vi "WL_XNET_GetDBCInfo.vi"(8 "err in":errorcluster caption="error") -> (0 "err out":errorcluster caption="error", 3 "DBC Settings":T1={"ByteOrder"=[enum."Motorola", enum."Motorola"], "Type"=[], "Factor"=[1.0, 1.0], "Offset"=[0.0, 0.0], "Startbit"=[27, 43], "Length"=[16, 16], "Mux"=[FALSE, FALSE], "Name"=["", ""]} {"Offset" format="%.3f"; "Factor" format="%.3f"})   [LabVIEW 2021]
uses:
  <vilib>/xnet/xnet.llb/XNET Database Close (Signal).vi
  <vilib>/xnet/xnet.llb/XNET Database Close (Cluster).vi
  <vilib>/xnet/xnet.llb/XNET Database Close (Database).vi
  WL_XNET_Globals.vi
  <resource>/objmgr/xnet.rc
panel:
  out "MuxDynamic":bool[](array[boolean])
  out "Mux":bool[](array[boolean])
  in  "default baud rate (0)":u64=500000
  in  "CAN DBC":path=path "G:/07_GLOBE/00_git/XLP80/02_Documentation/Daten Albert_10-08-2022/Globe_CAN_500_2022-08-08_v26.dbc"
  out "Frame":string[](array[string])
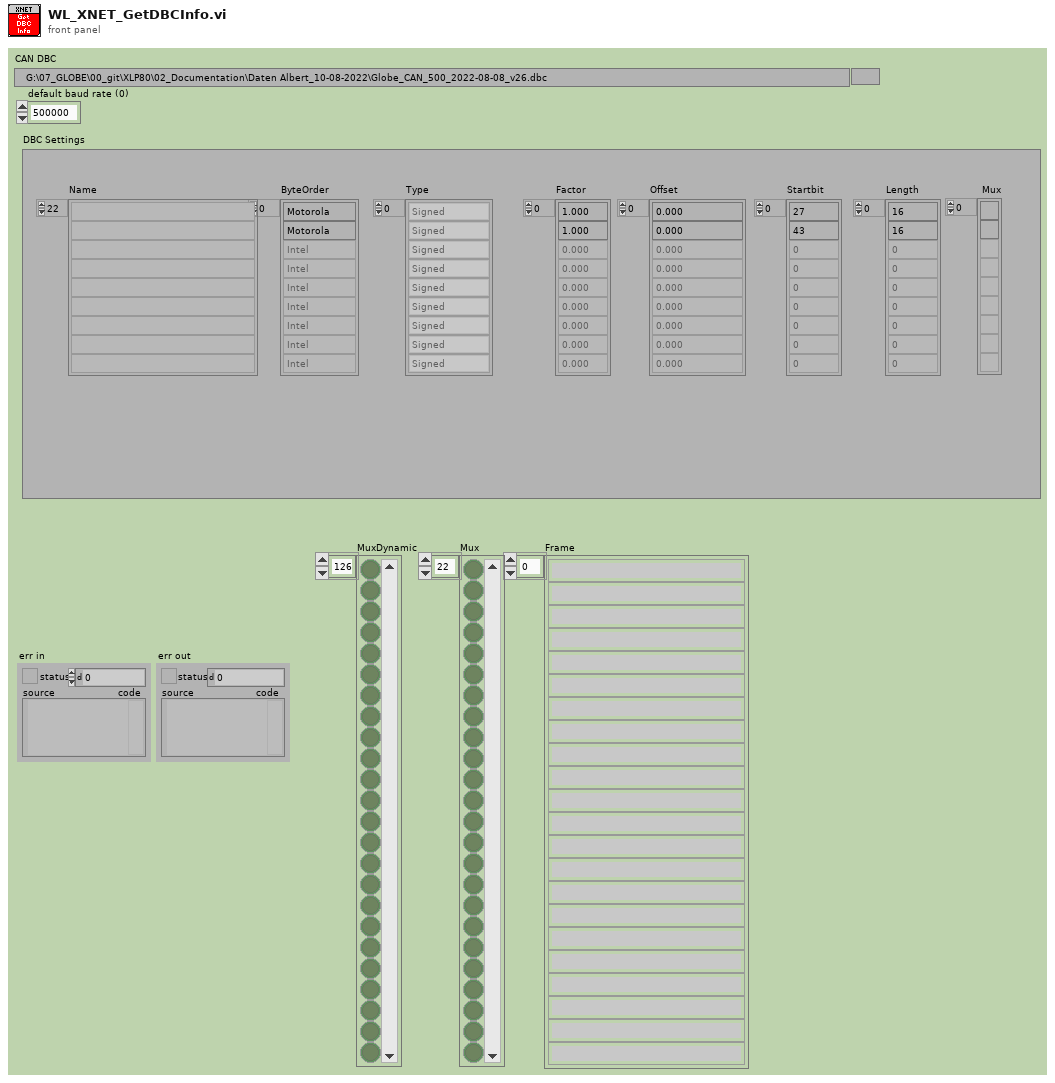
[diagram p1: front panel]
types:
  T1 = cluster{"ByteOrder":enum16{"Intel", "Motorola"}[], "Type":enum16{"Signed", "Unsigned", "IEEE Float", "Byte Array"}[], "Factor":dbl[], "Offset":dbl[], "Startbit":u32[], "Length":u32[], "Mux":bool[], "Name":string[]}
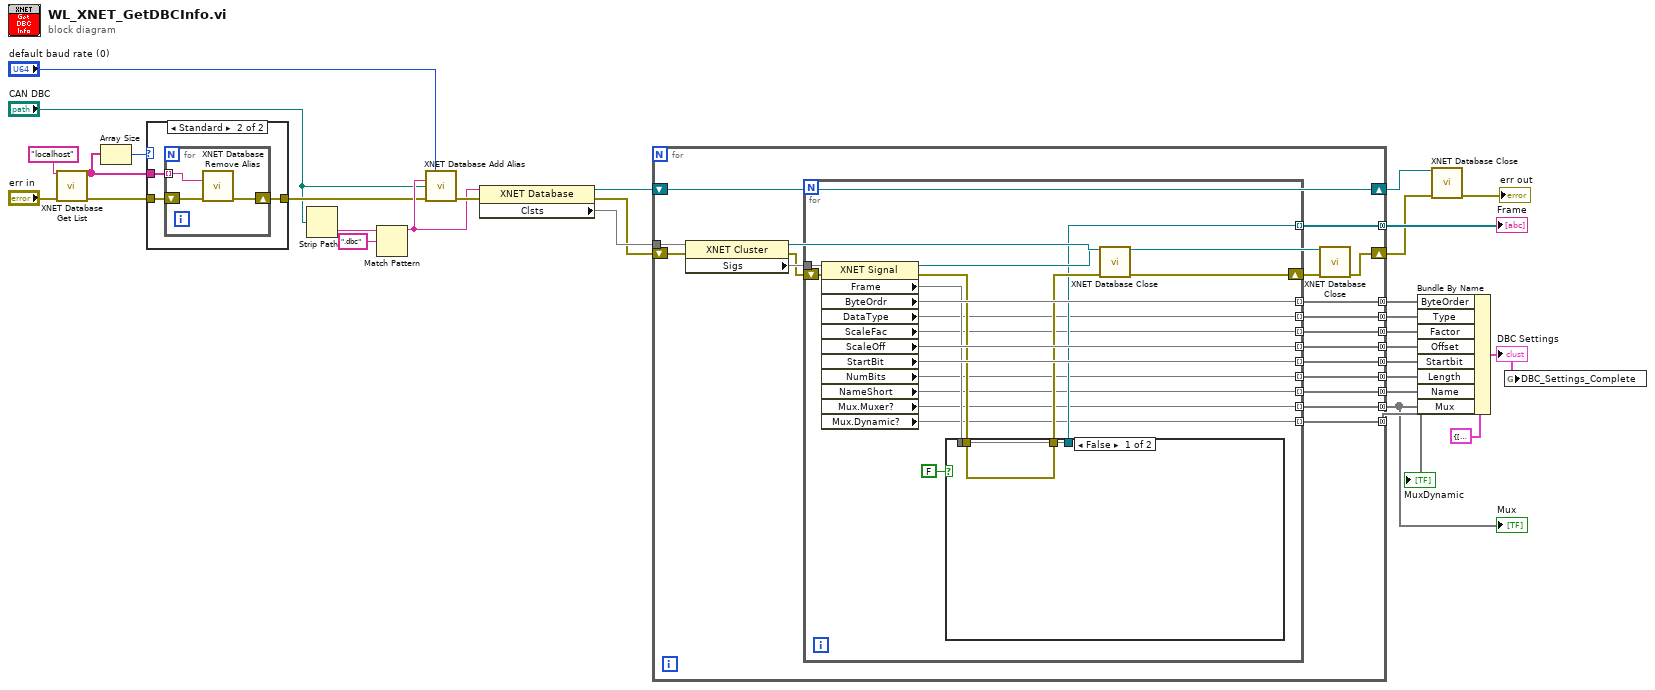
[diagram p0: block diagram]
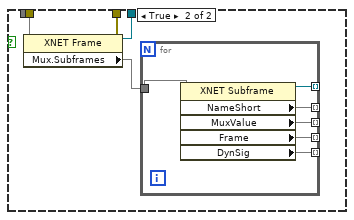
[diagram p3: hidden frame]
diagram:
  n1 = call <vilib>:"XNET Database Get List.vi"("IP address (localhost)"="localhost", "error in (no error)"="err in") -> ("array of alias"=w20:string[], "error out"=w22:errorcluster)  [unwired: 11 in, 1 out]
  n2 = Array Size(array=w20) -> (size(s)=w19:i32)
  n3 = case shown="Standard" w19 {
    tunnel: w22 -> [w31 w34]
    tunnel: [w31 w33] -> w21
    tunnel: w20 -> [_ w32]
    frame 0 {
    }
    frame Default {
      n4 = for {
        shift-right: [w36] -> w33
        shift-left: w34 -> [w37]
        tunnel: w32 -> [w35] mode=indexing
        n5 = call <vilib>:"XNET Database Remove Alias.vi"("alias"=w35, "error in (no error)"=w37) -> ("error out"=w36:errorcluster)  [unwired: 13 in]
      }
    }
  }
  n6 = Strip Path(path="CAN DBC") -> (name=w25:string)  [unwired: 1 out]
  n7 = Match Pattern(string=w25, regular expression=".dbc") -> (before substring=w24:string)  [unwired: 1 in, 3 out]
  n8 = call <vilib>:"XNET Database Add Alias.vi"("default baud rate (0)"="default baud rate (0)", "alias"=w24, "filepath"="CAN DBC", "error in (no error)"=w21) -> ("error out"=w27:errorcluster)  [unwired: 11 in]
  n9 = property class="XNET Database"(reference=w24, error in=w27) -> (reference out=w29:refnum<k21>, error out=w18:errorcluster, "Clsts"=w30)
  n10 = for {
    tunnel: w30 -> [w55]
    shift-right: [w48] -> w3
    shift-left: w29 -> [w48]
    tunnel: [w53] -> w9 mode=concatenating
    tunnel: [w52] -> w10 mode=concatenating
    tunnel: [w51] -> w12 mode=concatenating
    tunnel: [w50] -> w28 mode=concatenating
    tunnel: [w49] -> w13 mode=concatenating
    shift-right: [w45] -> w4
    shift-left: w18 -> [w47]
    tunnel: [w42] -> w8 mode=concatenating
    tunnel: [w41] -> w14 mode=concatenating
    tunnel: [w40] -> w11 mode=concatenating
    tunnel: [w39] -> w7 mode=concatenating
    tunnel: [w38] -> w6 mode=concatenating
    n11 = property class="XNET Cluster"(reference=w55, error in=w47) -> (reference out=w46:refnum<k21>, error out=w44:errorcluster, "Sigs"=w54)
    n12 = for {
      tunnel: w54 -> [w73]
      tunnel: [w72] -> w53 mode=indexing
      tunnel: [w71] -> w52 mode=indexing
      tunnel: [w59] -> w51 mode=indexing
      tunnel: [w63] -> w50 mode=indexing
      tunnel: [w67] -> w49 mode=indexing
      shift-right: [w69] -> w43
      shift-left: w44 -> [w70]
      tunnel: [w62] -> w42 mode=indexing
      tunnel: [w60] -> w41 mode=indexing
      tunnel: [w58] -> w40 mode=indexing
      tunnel: [w57] -> w39 mode=indexing
      tunnel: [w56] -> w38 mode=indexing
      n13 = property class="XNET Signal"(reference=w73, error in=w70) -> (reference out=w68:refnum<k21>, error out=w65:errorcluster, "Frame"=w66, "ByteOrdr"=w67, "DataType"=w59, "ScaleFac"=w58, "ScaleOff"=w71, "StartBit"=w72, "NumBits"=w62, "NameShort"=w57, "Mux.Muxer?"=w56, "Mux.Dynamic?"=w60)
      n14 = case shown="False" FALSE {
        tunnel: w66 -> [w74 w80]
        tunnel: [w74 w77] -> w63
        tunnel: w65 -> [w75 w79]
        tunnel: [w75 w78] -> w64
        frame False {
        }
        frame True {
          n15 = property class="XNET Frame"(reference=w80, error in=w79) -> (reference out=w77:refnum<k21>, error out=w78:errorcluster, "Mux.Subframes"=w76)
          n16 = for {
            tunnel: w76 -> [w86]
            tunnel: [w85] -> _ mode=indexing
            tunnel: [w84] -> _ mode=indexing
            tunnel: [w83] -> _ mode=indexing
            tunnel: [w82] -> _ mode=indexing
            tunnel: [w81] -> _ mode=indexing
            n17 = property class="XNET Subframe"(reference=w86) -> (reference out=w81:refnum<k21>, "NameShort"=w85, "MuxValue"=w84, "Frame"=w83, "DynSig"=w82)  [unwired: 1 in, 1 out]
          }
        }
      }
      n18 = call-poly <vilib>:"XNET Database Close.vi"("signal in"=w68, "error in (no error)"=w64) -> ("error out"=w69:errorcluster)  [unwired: 13 in]
    }
    n19 = call-poly <vilib>:"XNET Database Close.vi"("cluster in"=w46, "error in (no error)"=w43) -> ("error out"=w45:errorcluster)  [unwired: 13 in]
  }
  "Frame" <- w28
  "Mux" <- w6
  "MuxDynamic" <- w14
  n20 = Bundle By Name(cluster=T1 {"ByteOrder"=[], "Type"=[], "Factor"=[], "Offset"=[], "Startbit"=[], "Length"=[], "Mux"=[], "Name"=[]} ("DBC Settings"), "ByteOrder"=w13, "Type"=w12, "Factor"=w11, "Offset"=w10, "Startbit"=w9, "Length"=w8, "Name"=w7, "Mux"=w6) -> (w1:T1)
  "DBC Settings" <- w1
  n21 = call-poly <vilib>:"XNET Database Close.vi"("database in"=w3, "error in (no error)"=w4) -> ("error out"=→"err out":errorcluster)  [unwired: 13 in]
  n22 = global write "WL_XNET_Globals.vi" "DBC_Settings_Complete"(w1) -> ()
